vi "task.script_lua.vi"(5 "LuaVIEW reference":T1) -> (15 "error out":errorcluster)   [LabVIEW 2012]
doc: "Return the main script of the current task as a string. Useful for having a task log itself so that the script that actually ran, instead of a potentially modified script, can be reviewed later.\nResults:\nstr:script\nErrors:\nFunction must be called from a task context but was not."
uses:
  typedefs/t_LuaVIEW Reference.ctl
  typedefs/t_LuaVIEW Task State Methods.ctl
  subvis/private/LuaVIEW Push (string).vi
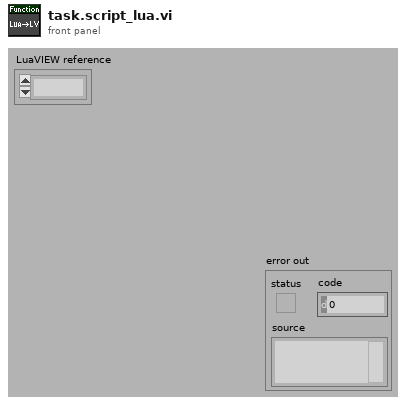
[diagram p1: front panel]
types:
  T1 = typedef "t_LuaVIEW Reference.ctl" = refnum<k1>
  T2 = typedef "t_LuaVIEW Task State Methods.ctl" = enum16{"cleanup", "set initial", "set mode", "set active mode", "set error", "get task info", "get script info", "set signal", "clear signal", "test handled", "test delegated", "test signal", "handle signal", "delegate signal", "allow signal", "disallow signal", "disallow all", "signals?", "delegated signals?", "protection++", "protection--", "protection=0", "message", "next message", "pop message", "message available?", "force stop", "set swap preps", "apply swap preps"}
  T3 = typedef "t_LuaVIEW Task State Pane.ctl" = refnum<vi>
  T4 = typedef "LuaVIEW Script Info.ctl" = cluster{"path":path, "description":string, "text":string, "parent index":i32, "version":string}
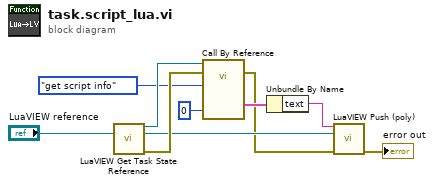
[diagram p0: block diagram]
diagram:
  n1 = call "LuaVIEW Get Task State Reference.vi"("LuaVIEW reference in"="LuaVIEW reference") -> ("task state reference"=w8:T3, "LuaVIEW reference out"=w6:T1, "error out"=w7:errorcluster)  [unwired: 12 in]
  n2 = call-by-ref "?"(reference=w8, error in=w7, "method"=t_LuaVIEW_Task_State_Methods."get script info", "script index"=0) -> (error out=w1:errorcluster, "script info"=w3:T4)  [unwired: 9 in, 5 out]
  n3 = Unbundle By Name(w3) -> ("text"=w2:string)
  n4 = call-poly "LuaVIEW Push (poly).vi"("string"=w2, "LuaVIEW reference in"=w6, "error in (no error)"=w1) -> ("error out"=→"error out":errorcluster)  [unwired: 11 in, 1 out]
